vi "Check-controls-for-conflicts.vi"(8 "error in (no error)":errorcluster, 10 "Data ref. in":refnum<data-value>, 11 "UI ref. in":refnum<data-value>) -> (0 "error out":errorcluster, 2 "Data ref.":refnum<data-value>, 3 "UI ref.":refnum<data-value>)   [LabVIEW 2013, in "CameraVision.lvlib" / "CV-UI.lvclass"]
uses:
  CV-UI.lvclass
  Main/CV-Main.lvclass
  CV-UI.lvclass/CV-UI.ctl
  Main/CV-Main.lvclass/CV-Main.ctl
  Main/Read Acquis params.vi
  Main/Read Config params.vi
  Main/Read Analysis params.vi
  Main/Read Temperature params.vi
  Read Control refs.vi
  Main/Acquisition/CV-Acquisition.lvclass
  Main/Configuration/CV-Configuration.lvclass
  Main/Analysis/CV-Analysis.lvclass
  Main/Temperature/CV-Temperature.lvclass
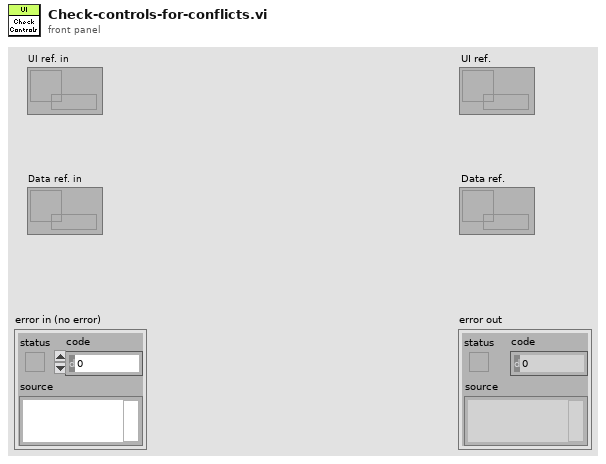
[diagram p1: front panel]
types:
  T1 = typedef "CameraVision.lvlib/CV-UI.lvclass/Control-names.ctl" = enum16{"Start acquisition", "Activate", "Stop acquisition", "Settings type", "Load settings", "Save settings", "Import images", "Camera selector", "Image type selector", "Batch browser", "Image refresh", "Parameter tabs", "Displays", "Processing tabs", "Processing selector", "Map characteristic", "Show info", "Manual trigger"}
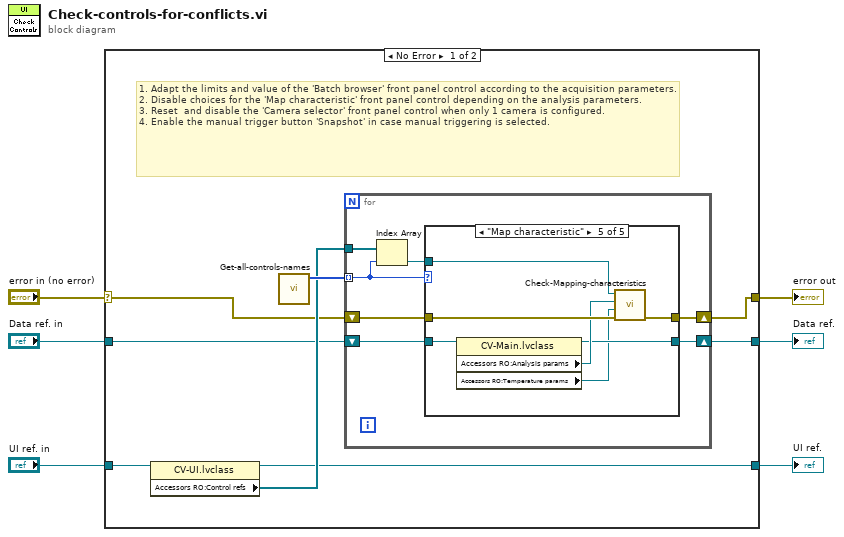
[diagram p0: block diagram]
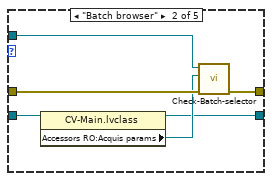
[diagram p3: hidden frame]
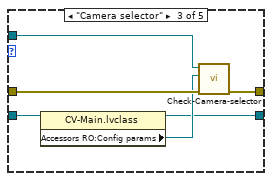
[diagram p4: hidden frame]
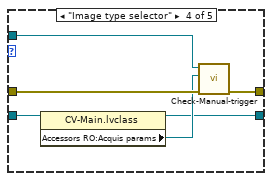
[diagram p5: hidden frame]
diagram:
  n1 = case shown="No Error" "error in (no error)" {
    selector: "error in (no error)" -> [w11 w51]
    tunnel: [w9 w51] -> w5
    tunnel: "UI ref. in" -> [w10 w50]
    tunnel: [w7 w50] -> w3
    tunnel: "Data ref. in" -> [w12 w49]
    tunnel: [w8 w49] -> w1
    frame No Error {
      # "1. Adapt the limits and value of the 'Batch browser' front panel control according to the acquisition parameters.\n2. Disable choices for the 'Map characteristic' front panel control depending on the analysis parameters.\n3. Reset  and disable the 'Camera selector' front panel control when only 1 camera is configured.\n4. Enable the manual trigger button 'Snapshot' in case manual triggering is selected."
      n2 = property class="CV-UI.lvclass"(reference=w10) -> (reference out=w7:refnum<data-value>, "Accessors RO:Control refs"=w13:refnum<vi>[])  [unwired: 1 in, 1 out]
      n3 = call "Get-all-controls-names.vi"() -> ("Controls"=w14:T1[])  [unwired: 11 in]
      n4 = for {
        tunnel: w14 -> [w19] mode=indexing
        tunnel: w13 -> [w21]
        shift-right: [w15] -> w8
        shift-left: w12 -> [w18]
        shift-right: [w16] -> w9
        shift-left: w11 -> [w17]
        n5 = Index Array(array=w21, index=w19) -> (element=w20:refnum<vi>)
        n6 = case shown="\"Map characteristic\"" w19 {
          tunnel: w20 -> [_ w26 w32 w38 w45]
          tunnel: w18 -> [w22 w29 w35 w41 w48]
          tunnel: w17 -> [w23 w28 w34 w40 w47]
          tunnel: [w23 w27 w33 w39 w46] -> w16
          tunnel: [w22 w24 w30 w36 w43] -> w15
          frame Default {
          }
          frame "Batch browser" {
            n7 = property class="CV-Main.lvclass"(reference=w29) -> (reference out=w24:refnum<data-value>, "Accessors RO:Acquis params"=w25:refnum<data-value>)  [unwired: 1 in, 1 out]
            n8 = call "Check-Batch-selector.vi"("error in"=w28, "Acquis. params. ref."=w25, "Batch browser"=w26) -> ("error IO"=w27:errorcluster)  [unwired: 5 in, 3 out]
          }
          frame "Camera selector" {
            n9 = property class="CV-Main.lvclass"(reference=w35) -> (reference out=w30:refnum<data-value>, "Accessors RO:Config params"=w31:refnum<data-value>)  [unwired: 1 in, 1 out]
            n10 = call "Check-Camera-selector.vi"("error in"=w34, "Config. params. ref."=w31, "Camera selector"=w32) -> ("error IO"=w33:errorcluster)  [unwired: 8 in]
          }
          frame "Image type selector" {
            n11 = property class="CV-Main.lvclass"(reference=w41) -> (reference out=w36:refnum<data-value>, "Accessors RO:Acquis params"=w37:refnum<data-value>)  [unwired: 1 in, 1 out]
            n12 = call "Check-Manual-trigger.vi"("error in"=w40, "Acquis. params. ref."=w37, "Manual trigger in"=w38) -> ("error IO"=w39:errorcluster)  [unwired: 8 in]
          }
          frame "Map characteristic" {
            n13 = property class="CV-Main.lvclass"(reference=w48) -> (reference out=w43:refnum<data-value>, "Accessors RO:Analysis params"=w44:refnum<data-value>, "Accessors RO:Temperature params"=w42:refnum<data-value>)  [unwired: 1 in, 1 out]
            n14 = call "Check-Mapping-characteristics.vi"("error in"=w47, "Temp. params. ref."=w42, "Analysis params. ref."=w44, "Map characteristics"=w45) -> ("error IO"=w46:errorcluster)  [unwired: 7 in]
          }
        }
      }
    }
    frame Error {
    }
  }
  "error out" <- w5
  "UI ref." <- w3
  "Data ref." <- w1
